vi "Attack.vi"(9 "Attack?":T1, 10 "Team Index":i32, 11 "View":i32[](array[numeric])) -> (0 "Enemy":i32, 1 "Direction":i32, 2 "Action":T2, 3 "View":i32[](array[numeric]), 4 "Enemy Found?":bool, 6 "Enemy Direction":i32)   [LabVIEW 2020, in "Common.lvlib"]
uses:
  Common.lvlib
  Type Defs/Action Enum.ctl
  Attack Options.ctl
  Type Defs/SB Type Defs.lvlib
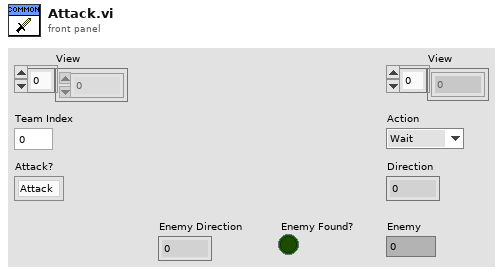
[diagram p1: front panel]
types:
  T1 = typedef "Common.lvlib/Attack Options.ctl" = enum16{"Attack", "Run", "Distract"}
  T2 = typedef "SB Type Defs.lvlib/Action Enum.ctl" = enum16{"Wait", "Move", "Attack", "Replicate"}
  T3 = typedef "SB Type Defs.lvlib/Direction Enum.ctl" = enum16{"NW", "N", "NE", "E", "SE", "S", "SW", "W"}
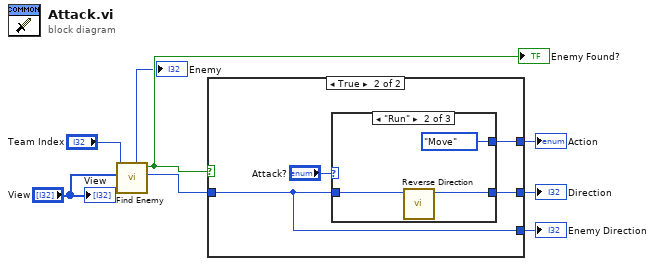
[diagram p0: block diagram]
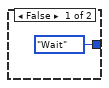
[diagram p2: hidden frame]
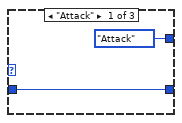
[diagram p3: hidden frame]
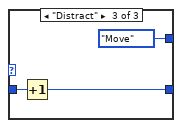
[diagram p4: hidden frame]
diagram:
  n1 = call "Find Enemy.vi"("View"="View", "Team Index"="Team Index") -> ("Direction"=w5:T3, "Found Enemy?"=w2:bool, "Enemy"=→"Enemy":i32)  [unwired: 7 in]
  "Enemy Found?" <- w2
  n2 = case shown="True" w2 {
    tunnel: [Action_Enum."Wait" ("Action") w13] -> w7
    tunnel: [_ w11] -> w8
    tunnel: [_ w10] -> w6
    tunnel: w5 -> [_ w10]
    frame False {
    }
    frame True {
      n3 = case shown="\"Run\"" "Attack?" {
        tunnel: [Action_Enum."Attack" ("Action") Action_Enum."Move" ("Action") Action_Enum."Move" ("Action")] -> w13
        tunnel: [w14 w16 w19] -> w11
        tunnel: w10 -> [w14 w17 w20]
        frame "Attack" {
        }
        frame "Run" {
          n4 = call "Reverse Direction.vi"("Direction in"=w17) -> ("Reverse Direction"=w16:i32)  [unwired: 10 in]
        }
        frame "Distract" {
          n5 = Increment(x=w20) -> (x+1=w19:T3)
        }
      }
    }
  }
  "Action" <- w7
  "Direction" <- w8
  "Enemy Direction" <- w6
  "View" <- "View"
